vi "DevMode.vi"(8 "error in (no error)":errorcluster, 9 "Compile Locally":refnum<vi>, 11 "path":path) -> (0 "error out":errorcluster, 2 "Student":bool, 3 "Dev Machine":bool)   [LabVIEW 2014]
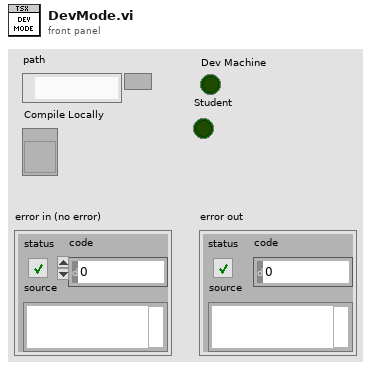
[diagram p1: front panel]
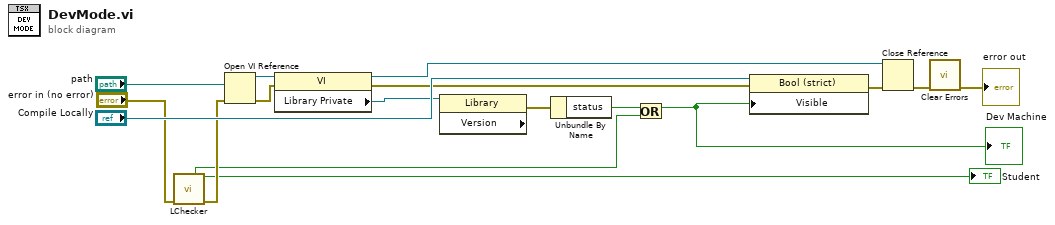
[diagram p0: block diagram]
diagram:
  n1 = call "LChecker.vi"("error in (no error)"="error in (no error)") -> ("DevMode"=w2:bool, "Student"=→"Student":bool, "error out"=w4:errorcluster)  [unwired: 12 in]
  n2 = Open VI Reference(vi path="path", error in (no error)=w4) -> (vi reference=w17:refnum<vi>, error out=w16:errorcluster)  [unwired: 4 in]
  n3 = property class="VI"(reference=w17, error in=w16) -> (reference out=w14:refnum<vi>, error out=w12:errorcluster, "Library Private"=w11:refnum<vi>)
  n4 = property class="Library" props=["Version"](reference=w11) -> (error out=w10:errorcluster)  [unwired: 1 in, 2 out]
  n5 = Unbundle By Name(w10) -> ("status"=w9:bool)
  n6 = Or(x=w9, y=w2) -> (x .or. y?=w3:bool)
  "Dev Machine" <- w3
  n7 = property class="Bool (strict)"(reference="Compile Locally", error in=w12, "Visible"=w3) -> (error out=w8:errorcluster)  [unwired: 1 out]
  n8 = Close Reference(reference=w14, error in (no error)=w8) -> (error out=w7:errorcluster)
  n9 = call <vilib>:"Clear Errors.vi"("error in (no error)"=w7) -> ("error out"=→"error out":errorcluster)  [unwired: 5 in, 1 out]
